vi "Datadashboard CD RT Driver VI.vi"(7 "Operation":T1, 11 "Device Reference in":T2 format="%.0x") -> (0 "Error Code":i32)   [LabVIEW 2013, in "Datadashboard CD Custom Device.lvlib"]
uses:
  Datadashboard CD Custom Device.lvlib
  <vilib>/NI Veristand/Custom Device API/Custom Device Item Ref.ctl
  <vilib>/NI Veristand/Custom Device API/Hardware Interface Driver VI Operation.ctl
  <vilib>/NI Veristand/Custom Device API/Data Access Type.ctl
  <vilib>/NI Veristand/Custom Device API/Global Data Refs.vi
  <vilib>/NI Veristand/Custom Device API/Data Reference.ctl
  <vilib>/lvdsc/NI_DSC.lvlib
  <vilib>/NI Veristand/Custom Device API/Custom Device API.lvlib
  <vilib>/NI Veristand/Custom Device API/Custom Device Channel Type.ctl
  Channel Block Ref.ctl
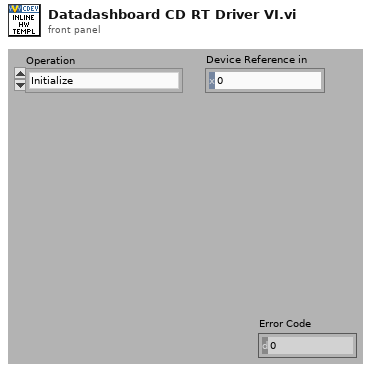
[diagram p1: front panel]
types:
  T1 = typedef "Custom Device API.lvlib/Hardware Interface Driver VI Operation.ctl" = enum16{"Initialize", "Start", "Read Data from HW", "Write Data to HW", "Close"}
  T2 = typedef "Custom Device API.lvlib/Custom Device Item Ref.ctl" = u64
  T3 = typedef "Channel Block Ref.ctl" = cluster{"error":errorcluster, "Values Read":dbl[], "Values Array Write":dbl[], "Dep. Channel Refs":T2[], "shared variables out":refnum<k21>[], "Channel Data Reference":T4[]}
  T4 = typedef "Custom Device API.lvlib/Data Reference.ctl" = i32
  T5 = typedef "Custom Device API.lvlib/Data Access Type.ctl" = enum16{"Read", "Write"}
  T6 = typedef "Custom Device API.lvlib/Custom Device Channel Type.ctl" = enum16{"Input", "Output"}
  T7 = enum16{"Read", "Write", "ReadWrite", "BufferedRead", "BufferedReadWrite"}
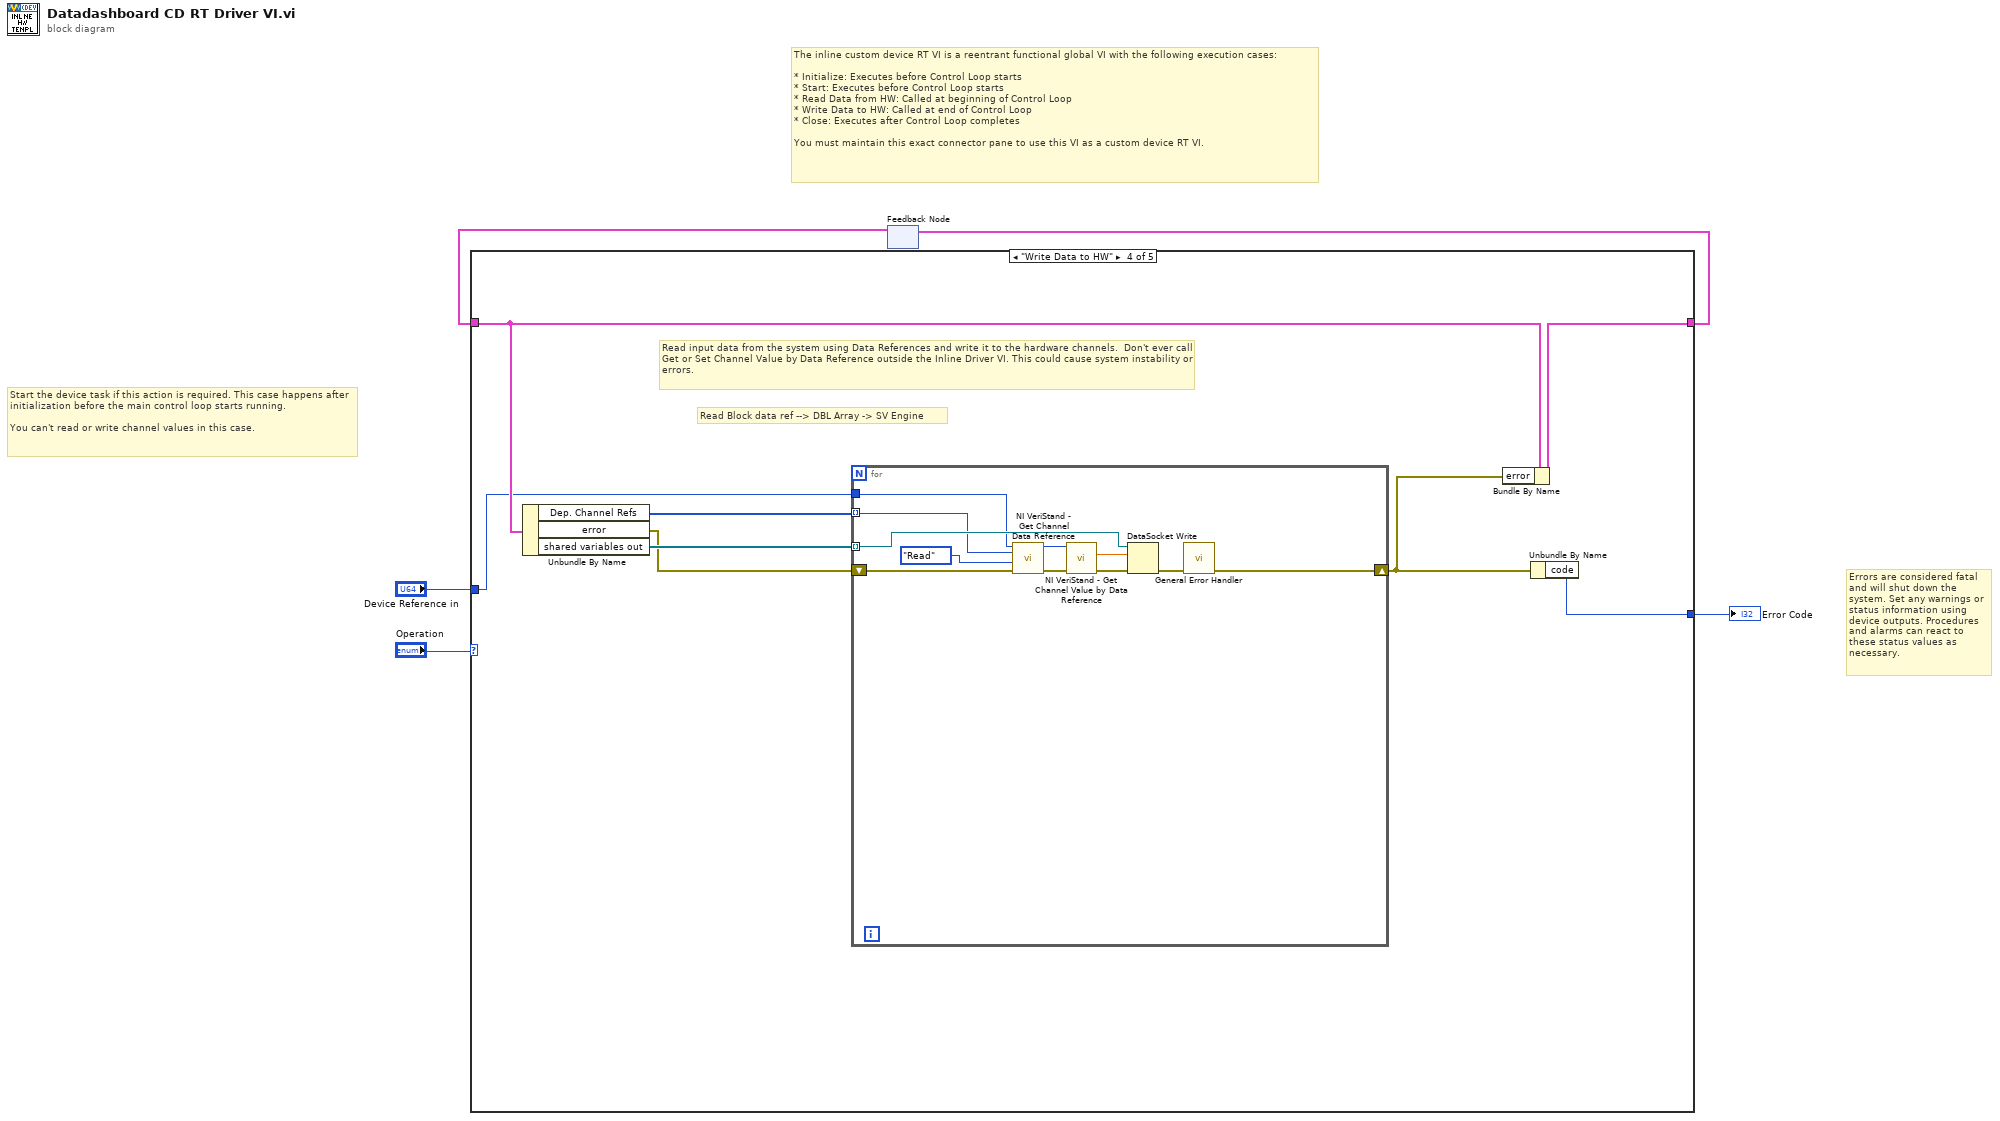
[diagram p0: block diagram]
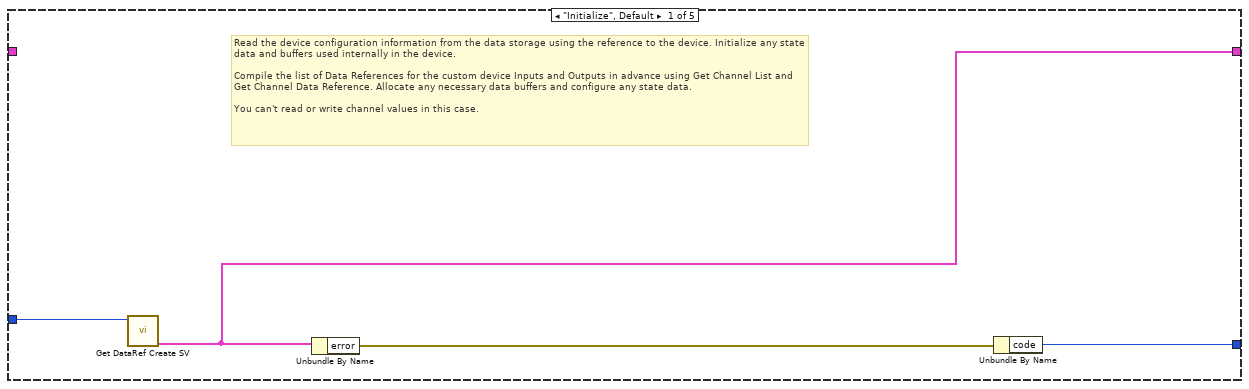
[diagram p2: hidden frame]
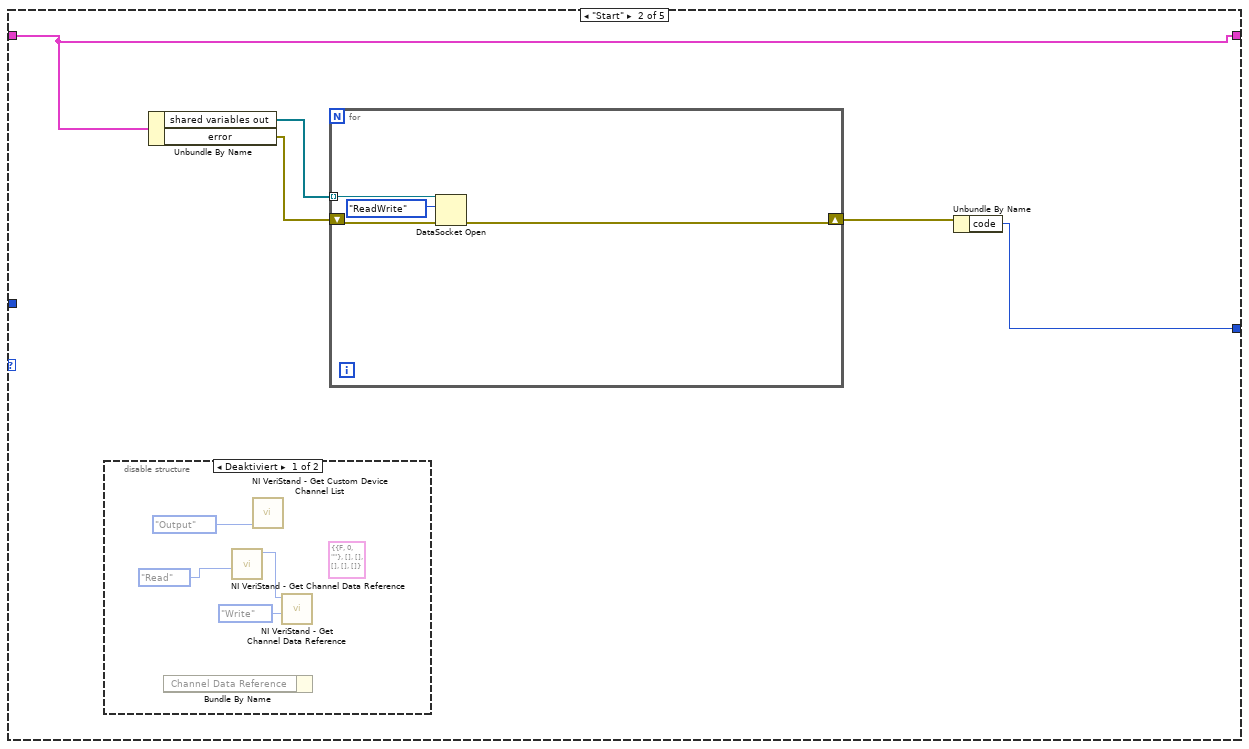
[diagram p3: hidden frame]
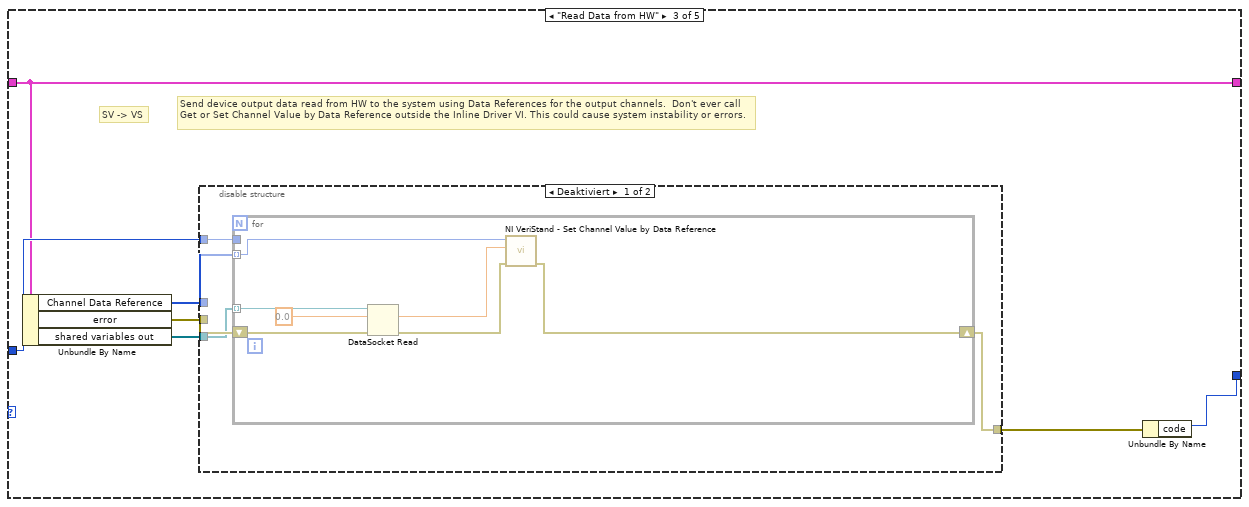
[diagram p5: hidden frame]
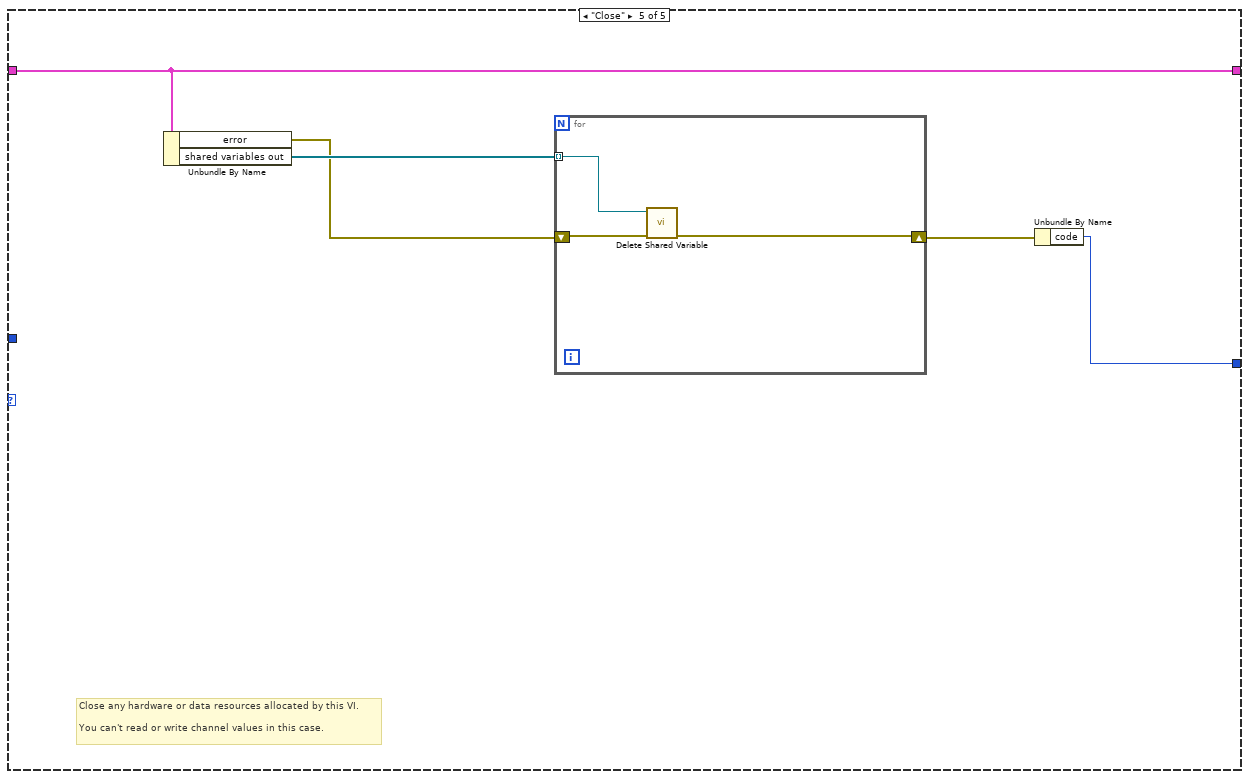
[diagram p7: hidden frame]
diagram:
  # "Start the device task if this action is required. This case happens after initialization before the main control loop starts running.\n\nYou can't read or write channel values in this case."
  # "Errors are considered fatal and will shut down the system. Set any warnings or status information using device outputs. Procedures and alarms can react to these status values as necessary."
  # "The inline custom device RT VI is a reentrant functional global VI with the following execution cases:\n\n* Initialize: Executes before Control Loop starts\n* Start: Executes before Control Loop starts\n* Read Data from HW: Called at beginning of Control Loop\n* Write Data to HW: Called at end of Control Loop\n* Close: Executes after Control Loop completes\n\nYou must maintain this exact connector pane to use this VI as a custom device RT VI."
  n1 = feedback #1() -> (w3:T3)  [unwired: 1 out]
  n2 = case shown="\"Write Data to HW\"" "Operation" {
    tunnel: [w6 w10 w23 w48 w65] -> w4
    tunnel: w3 -> [_ w10 w23 w49 w65]
    tunnel: "Device Reference in" -> [w8 _ w24 w42 _]
    tunnel: [w9 w11 w29 w47 w61] -> w1
    frame "Initialize", Default {
      # "Read the device configuration information from the data storage using the reference to the device. Initialize any state data and buffers used internally in the device.\n\nCompile the list of Data References for the custom device Inputs and Outputs in advance using Get Channel List and Get Channel Data Reference. Allocate any necessary data buffers and configure any state data.\n\nYou can't read or write channel values in this case."
      n3 = call "Get DataRef Create SV.vi"("Device Ref in"=w8) -> ("Ausgangs-Cluster"=w6:T3)  [unwired: 10 in]
      n4 = Unbundle By Name(w6) -> ("error"=w7:errorcluster)
      n5 = Unbundle By Name(w7) -> ("code"=w9:i32)
    }
    frame "Start" {
      n6 = disable-structure shown="Deaktiviert" {
        frame Disabled {
          (unwired) T3 {"error"={"status"=FALSE, "code"=0, "source"=""}, "Values Read"=[], "Values Array Write"=[], "Dep. Channel Refs"=[], "shared variables out"=[], "Channel Data Reference"=[]} ("Ausgangs-Cluster")
          n7 = Bundle By Name() -> ()  [unwired: 2 in, 1 out]
          n8 = call <vilib>:"NI VeriStand - Get Channel Data Reference.vi"("Access"=Data_Access_Type."Read") -> ("Device Ref out"=w17:T2)  [unwired: 8 in, 2 out]
          n9 = call <vilib>:"NI VeriStand - Get Custom Device Channel List.vi"("Channel Type"=Custom_Device_Channel_Type."Output") -> ()  [unwired: 8 in, 3 out]
          n10 = call <vilib>:"NI VeriStand - Get Channel Data Reference.vi"("Access"=Data_Access_Type."Write", "Device Ref in"=w17) -> ()  [unwired: 7 in, 3 out]
        }
        frame Enabled {
        }
      }
      n11 = Unbundle By Name(w10) -> ("shared variables out"=w14:refnum<k21>[], "error"=w13:errorcluster)
      n12 = for {
        tunnel: w14 -> [w22] mode=indexing
        shift-right: [w20] -> w12
        shift-left: w13 -> [w21]
        n13 = DataSocket Open(8:w21, 10:T7."ReadWrite" ("Modus"), 11:w22) -> (0:w20:errorcluster)  [unwired: 1 in, 1 out]
      }
      n14 = Unbundle By Name(w12) -> ("code"=w11:i32)
    }
    frame "Read Data from HW" {
      # "SV -> VS"
      # "Send device output data read from HW to the system using Data References for the output channels.  Don't ever call Get or Set Channel Value by Data Reference outside the Inline Driver VI. This could cause system instability or errors."
      n15 = Unbundle By Name(w23) -> ("Channel Data Reference"=w27:T4[], "error"=w28:errorcluster, "shared variables out"=w25:refnum<k21>[])
      n16 = disable-structure shown="Deaktiviert" {
        disable-tunnel: w28 -> [w34 _]
        disable-tunnel: w27 -> [w33 _]
        disable-tunnel: [w32 _] -> w26
        disable-tunnel: w25 -> [w31 _]
        disable-tunnel: w24 -> [w30 _]
        frame Disabled {
          n17 = for {
            tunnel: w33 -> [w39] mode=indexing
            shift-right: [w38] -> w32
            shift-left: w34 -> [w40]
            tunnel: w31 -> [w41] mode=indexing
            tunnel: w30 -> [_]
            n18 = DataSocket Read(8:w40, 10:0.0, 11:w41) -> (0:w35:errorcluster, 2:w36:dbl)  [unwired: 2 in, 5 out]
            n19 = call <vilib>:"NI VeriStand - Set Channel Value by Data Reference.vi"("error in (no error)"=w35, "Value"=w36, "Data Reference in"=w39) -> ("error out"=w38:errorcluster)  [unwired: 8 in]
          }
        }
        frame Enabled {
        }
      }
      n20 = Unbundle By Name(w26) -> ("code"=w29:i32)
    }
    frame "Write Data to HW" {
      # "Read Block data ref --> DBL Array -> SV Engine"
      # "Read input data from the system using Data References and write it to the hardware channels.  Don't ever call Get or Set Channel Value by Data Reference outside the Inline Driver VI. This could cause system instability or errors."
      n21 = Unbundle By Name(w49) -> ("Dep. Channel Refs"=w43:T2[], "error"=w45:errorcluster, "shared variables out"=w46:refnum<k21>[])
      n22 = for {
        tunnel: w46 -> [w60] mode=indexing
        shift-right: [w59] -> w44
        shift-left: w45 -> [w53]
        tunnel: w43 -> [w54] mode=indexing
        tunnel: w42 -> [w50]
        n23 = call <vilib>:"NI VeriStand - Get Channel Data Reference.vi"("error in (no error)"=w53, "Access"=Data_Access_Type."Read", "Channel Ref in"=w54, "Device Ref in"=w50) -> ("error out"=w52:errorcluster, "Channel Data Reference"=w56:T4)  [unwired: 5 in, 1 out]
        n24 = call <vilib>:"NI VeriStand - Get Channel Value by Data Reference.vi"("error in (no error)"=w52, "Data Reference in"=w56) -> ("error out"=w51:errorcluster, "Value"=w55:dbl)  [unwired: 8 in]
        n25 = DataSocket Write(8:w51, 10:w55, 11:w60) -> (0:w58:errorcluster)  [unwired: 1 in, 2 out]
        n26 = call <vilib>:"General Error Handler.vi"("error in (no error)"=w58) -> ("error out"=w59:errorcluster)  [unwired: 10 in, 4 out]
      }
      n27 = Bundle By Name(cluster=w49, "error"=w44) -> (w48:T3)
      n28 = Unbundle By Name(w44) -> ("code"=w47:i32)
    }
    frame "Close" {
      # "Close any hardware or data resources allocated by this VI.\n\nYou can't read or write channel values in this case."
      n29 = Unbundle By Name(w65) -> ("error"=w63:errorcluster, "shared variables out"=w64:refnum<k21>[])
      n30 = for {
        tunnel: w64 -> [w67] mode=indexing
        shift-right: [w66] -> w62
        shift-left: w63 -> [w68]
        n31 = call <vilib>:"Delete Shared Variable.vi"("error in (no error)"=w68, "shared variable"=w67) -> ("error out"=w66:errorcluster)  [unwired: 9 in]
      }
      n32 = Unbundle By Name(w62) -> ("code"=w61:i32)
    }
  }
  "Error Code" <- w1
  n33 = feedback-in #1(w4) -> ()
